vi "ExerciceSerrure3.vi"() -> ()   [LabVIEW 2018]
uses:
  Serrure_Var.vi
panel:
  out "?":picture
  out "?":bool
  in  "?":bool
  out "Tentatives Max":dbl
  out "Tentatives":dbl
  in  "Code 3":i8(knob) min=0 max=9 scale=0.0..9.0
  in  "Code 2":i8(knob) min=0 max=9 scale=0.0..9.0
  in  "Code 1":i8(knob) min=0 max=9 scale=0.0..9.0
  # "/"
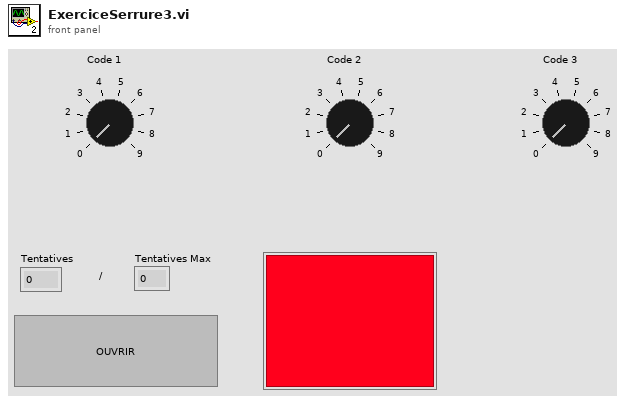
[diagram p1: front panel]
types:
  T1 = typedef "imagedata.ctl" = cluster{"image type":i32, "image depth":i32, "image":u8[], "mask":u8[], "colors":u32[], "Rectangle":cluster{"left":i16, "top":i16, "right":i16, "bottom":i16}}
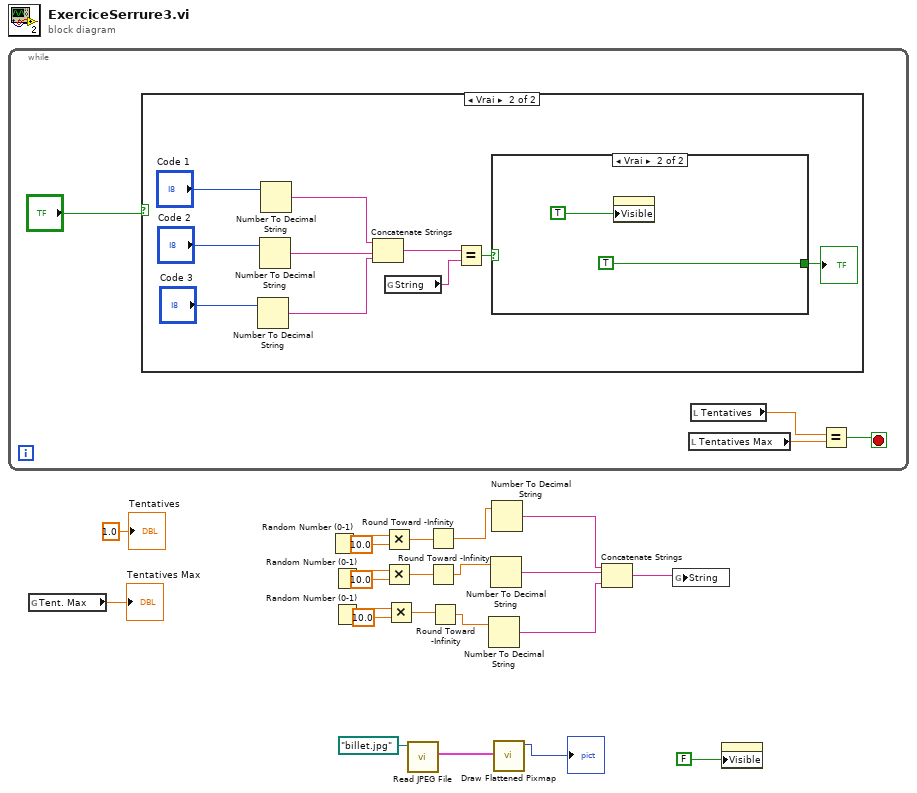
[diagram p0: block diagram]
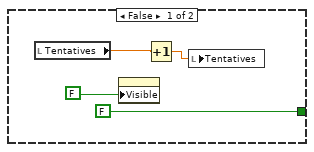
[diagram p3: hidden frame]
diagram:
  n1 = while {
    stop <- w26 stop-if-true
    n2 = case shown="Vrai" "?" {
      frame False {
      }
      frame True {
        n3 = Number To Decimal String(number="Code 3") -> (decimal integer string=w31:string)  [unwired: 1 in]
        n4 = Number To Decimal String(number="Code 2") -> (decimal integer string=w32:string)  [unwired: 1 in]
        n5 = Number To Decimal String(number="Code 1") -> (decimal integer string=w33:string)  [unwired: 1 in]
        n6 = Concatenate Strings(w33, w32, w31) -> (w30:string)
        n7 = global read "Serrure_Var.vi" "String"() -> (w29:string)
        n8 = Equal?(x=w30, y=w29) -> (x = y?=w28:bool)
        n9 = case shown="Vrai" w28 {
          tunnel: [FALSE TRUE] -> w27
          frame False {
            n10 = local read "Tentatives"() -> (w38:dbl)
            n11 = property class="Image"("Visible"=FALSE) -> ()  [unwired: 2 in, 2 out]
            n12 = Increment(x=w38) -> (x+1=w39:dbl)
            n13 = local write "Tentatives"(w39) -> ()
          }
          frame True {
            n14 = property class="Image"("Visible"=TRUE) -> ()  [unwired: 2 in, 2 out]
          }
        }
        "?" <- w27
      }
    }
    n15 = local read "Tentatives Max"() -> (w25:dbl)
    n16 = local read "Tentatives"() -> (w24:dbl)
    n17 = Equal?(x=w24, y=w25) -> (x = y?=w26:bool)
  }
  n18 = global read "Serrure_Var.vi" "Tent. Max"() -> (→"Tentatives Max":dbl)
  n19 = Random Number (0-1)() -> (number: 0 to 1=w16:dbl)
  n20 = Random Number (0-1)() -> (number: 0 to 1=w15:dbl)
  n21 = Random Number (0-1)() -> (number: 0 to 1=w14:dbl)
  n22 = Multiply(x=w16, y=10.0) -> (x*y=w10:dbl)
  n23 = Multiply(x=w15, y=10.0) -> (x*y=w9:dbl)
  n24 = Multiply(x=w14, y=10.0) -> (x*y=w8:dbl)
  n25 = call <vilib>:"Read JPEG File.vi"("path to JPEG file"=path "billet.jpg") -> ("image data"=w21:T1)  [unwired: 8 in, 2 out]
  n26 = Round Toward -Infinity(1:w10) -> (0:w7:dbl)
  n27 = Round Toward -Infinity(1:w9) -> (0:w6:dbl)
  n28 = Round Toward -Infinity(1:w8) -> (0:w5:dbl)
  n29 = Number To Decimal String(number=w5) -> (decimal integer string=w2:string)  [unwired: 1 in]
  n30 = Number To Decimal String(number=w6) -> (decimal integer string=w3:string)  [unwired: 1 in]
  n31 = Number To Decimal String(number=w7) -> (decimal integer string=w4:string)  [unwired: 1 in]
  n32 = call <vilib>:"Draw Flattened Pixmap.vi"("image data"=w21) -> ("new picture"=→"?":picture)  [unwired: 8 in]
  n33 = Concatenate Strings(w4, w3, w2) -> (w1:string)
  n34 = global write "Serrure_Var.vi" "String"(w1) -> ()
  n35 = property class="Image"("Visible"=FALSE) -> ()  [unwired: 2 in, 2 out]
  "Tentatives" <- 1.0 ("Tentatives")
